vi "LVClass_Pupil Write Data Pupil to txt file.vi"(0 "Pupil in":refnum<class "Pupil.lvclass">, 5 "file path (dialog if empty)":path, 7 "Data Pupil":u8[][](array[numeric]), 11 "error in (no error)":errorcluster) -> (4 "Pupil out":refnum<class "Pupil.lvclass">, 15 "error out":errorcluster)   [LabVIEW 2020, in "Pupil.lvclass"]
uses:
  Pupil.lvclass
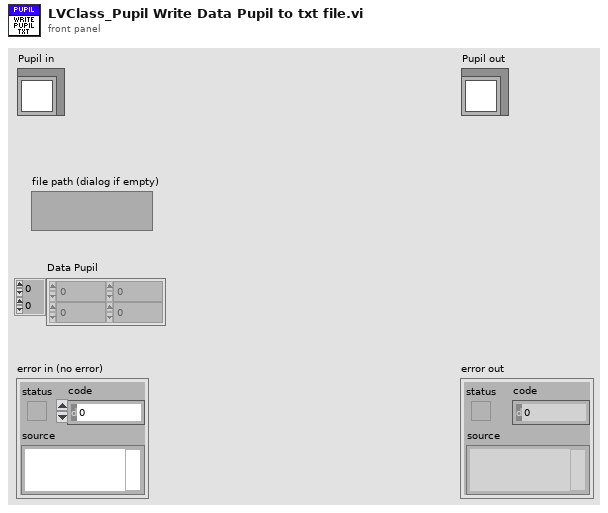
[diagram p1: front panel]
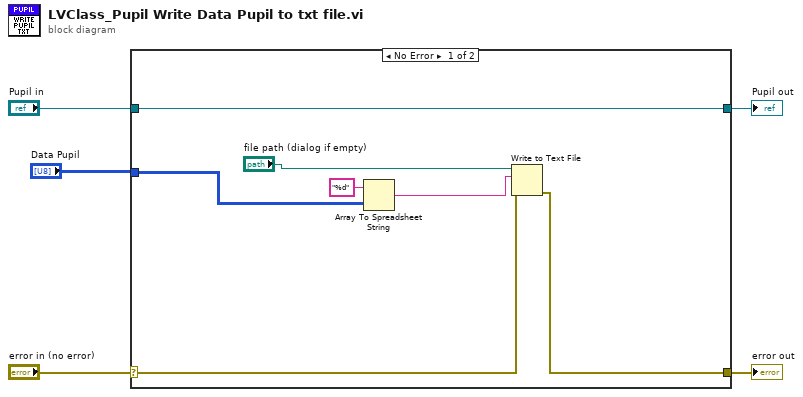
[diagram p0: block diagram]
diagram:
  n1 = case shown="No Error" "error in (no error)" {
    selector: "error in (no error)" -> [w7 w14]
    tunnel: [w6 w14] -> w4
    tunnel: [w12 w13] -> w2
    tunnel: "Pupil in" -> [w12 w13]
    tunnel: "Data Pupil" -> [w11 _]
    frame No Error {
      n2 = Array To Spreadsheet String(array=w11, 3:"%d" ("format string")) -> (spreadsheet string=w8:string)  [unwired: 1 in]
      n3 = Write to Text File(file (use dialog)="file path (dialog if empty)", text=w8, error in=w7) -> (error out=w6:errorcluster)  [unwired: 1 in, 2 out]
    }
    frame Error {
    }
  }
  "error out" <- w4
  "Pupil out" <- w2
